vi "Set Number of Servos.vi"(0 "Arduino Resource":T1={"VISA resource"="", "Board Type"=enum."Arduino Uno", "Connection Type"=enum."USB / Serial", "Bytes Per Packet (15)"=15}, 7 "Number Of Servos (1)":u8=1, 11 "error in":errorcluster) -> (4 "Arduino Resource":T1={"VISA resource"="", "Board Type"=enum."Arduino Uno", "Connection Type"=enum."USB / Serial", "Bytes Per Packet (15)"=15}, 15 "error out":errorcluster)   [LabVIEW 2011, in "LabVIEW Interface for Arduino.lvlib"]
doc: "Set Number of Servos creates memory space on the Arduino for the specified number of servos. This VI creates a zero indexed array of the specified number of servos. After calling this VI you can refer to each servo by number (starting with servo 0)."
uses:
  <vilib>/LabVIEW Interface for Arduino/LabVIEW Interface for Arduino.lvlib
  <vilib>/LabVIEW Interface for Arduino/Private/Type Defs/Arduino Resource.ctl
  <vilib>/LabVIEW Interface for Arduino/Private/Type Defs/Board Type.ctl
  <vilib>/LabVIEW Interface for Arduino/Private/Type Defs/Command.ctl
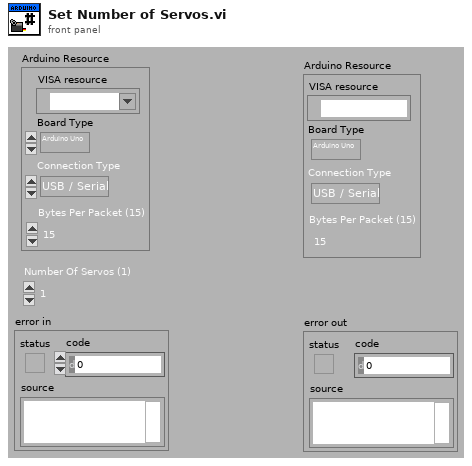
[diagram p1: front panel]
types:
  T1 = typedef "LabVIEW Interface for Arduino.lvlib/Arduino Resource.ctl" = cluster{"VISA resource":refnum<visa-resource-name>, "Board Type":T2, "Connection Type":enum8{"USB / Serial"}, "Bytes Per Packet (15)":u8}
  T2 = typedef "LabVIEW Interface for Arduino.lvlib/Board Type.ctl" = enum16{"Arduino Uno", "Dimuelanove w/Atmega 328", "Mega 2560", "Chipkit Uno32", "Chipkit Max32"}
  T3 = typedef "LabVIEW Interface for Arduino.lvlib/Command.ctl" = enum8{"setArduinoMode", "flushSerial", "setPinMode", "digitalWritePin", "digitalWritePort", "tone", "digitalReadPin", "digitalReadPort", "analogReadPin", "analogReadPort", "pwmWritePin", "pwmWritePort", "sevenSegment_Configure", "sevenSegment_Write", "I2C Init", "I2C Write", "I2C Read", "SPI Init", "SPI Set Bit Order", "SPI Set Clock Divider", "SPI Set Data Mode", "SPI Send / Receive", "SPI Close", "Servo Set Num Servos", "Servo Config Servo", "Servo Write Angle", "Servo Read Angle", "Servo Write Pulse Width", "Servo Read Pulse Width", "Servo Detach", "LCD Init", "LCD Set Size", "LCD Set Cursor Mode", "LCD Clear", "LCD Set Cursor Position", "LCD Print", "LCD Display Power", "LCD Scroll Display", "LCD Autoscroll", "LCD Print Direction", "LCD Create Custom Char", "LCD Print Custom Char", "contAcqOn", "contAcqOff", "getFirmwareVersion", "FiniteSampleStart"}
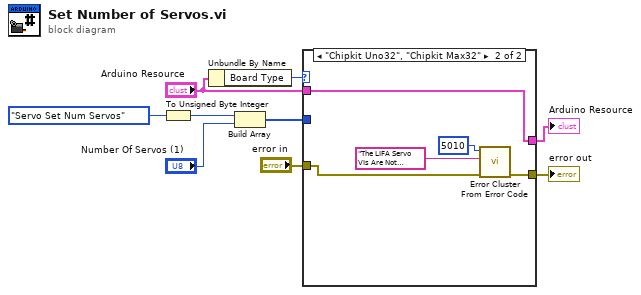
[diagram p0: block diagram]
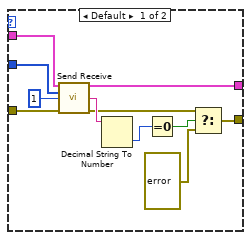
[diagram p2: hidden frame]
diagram:
  n1 = To Unsigned Byte Integer(number=Command."Servo Set Num Servos" ("Command")) -> (unsigned 8bit integer=w8:u8)
  n2 = Unbundle By Name("Arduino Resource") -> ("Board Type"=w1:T2)
  n3 = Build Array(w8, "Number Of Servos (1)") -> (w6:u8[])
  n4 = case shown="\"Chipkit Uno32\", \"Chipkit Max32\"" w1 {
    tunnel: [w11 w23] -> w3
    tunnel: w6 -> [w14 _]
    tunnel: "Arduino Resource" -> [w13 w22]
    tunnel: "error in" -> [w12 w21]
    tunnel: [w10 w22] -> w2
    frame Default {
      n5 = call <vilib>:"Send Receive.vi"("Arduino Resource"=w13, "Data"=w14, "Bytes To Read (0)"=u8 1, "error in"=w12) -> ("Arduino Resource"=w10:T1, "Read Buffer"=w16:string, "error out"=w15:errorcluster)  [unwired: 9 in]
      n6 = Decimal String To Number(string=w16) -> (number=w17:i32)  [unwired: 2 in, 1 out]
      n7 = Equal To 0?(x=w17) -> (x = 0?=w18:bool)
      n8 = Select(t=w15, s=w18, f=errorcluster {"status"=TRUE, "code"=5006, "source"="Unable to allocate memory on Arduino to store servo settings.  Please reset your Arduino and try running your program again.  If you continue to get this error try using fewer servos."}) -> (s? t:f=w11:errorcluster)
    }
    frame "Chipkit Uno32", "Chipkit Max32" {
      n9 = call <vilib>:"Error Cluster From Error Code.vi"("error in (no error)"=w21, "error message (\"\")"="The LIFA Servo VIs Are Not Supported On Chipkit Targets." ("source"), "error code (0)"=5010) -> ("error out"=w23:errorcluster)  [unwired: 6 in]
    }
  }
  "Arduino Resource" <- w2
  "error out" <- w3
